vi "Untitled 2.vi"() -> ()   [LabVIEW 2020]
uses:
  <vilib>/gpm_packages/@cs/linked-list/Source/Linked List/Linked List/Linked List.lvclass
  C:/Program Files/National Instruments/LabVIEW 2020/vi.lib/gpm_packages/@cs/linked-list/Source/Linked List/ILinkedList/ILinked List.lvclass
  <vilib>/gpm_packages/@cs/persistence/source/CAML/CAML.lvclass
  C:/Program Files/National Instruments/LabVIEW 2020/vi.lib/gpm_packages/@cs/persistence/source/IPersist/IPersist.lvclass
  <vilib>/gpm_packages/@cs/persistence/source/XML/XML.lvclass
  <vilib>/gpm_packages/@cs/user-manager/Source/User Configuration Manager/User Configuration Manager.lvclass
  <vilib>/gpm_packages/@cs/user-manager/Source/SHA-1 Encryption/SHA-1.lvclass
  C:/Program Files/National Instruments/LabVIEW 2020/vi.lib/gpm_packages/@cs/user-manager/Source/iEncryption/iEncryption.lvclass
  <vilib>/gpm_packages/@cs/persistence/source/IPersist/IPersist.lvclass
  68168d1c-9d56-4a75-be37-98398c79d179.vi
  <vilib>/gpm_packages/@cs/linked-list/Source/Linked List/ILinkedList/ILinked List.lvclass
  <vilib>/gpm_packages/@cs/linked-list/Source/Linked List/Linked List Ref/Linked List Ref.lvclass
panel:
  out "error out 2":errorcluster
  out "error out":errorcluster
  out "Verification Message":string
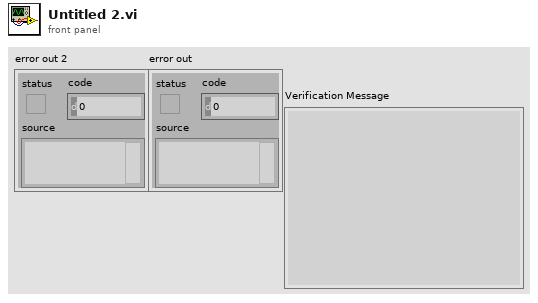
[diagram p1: front panel]
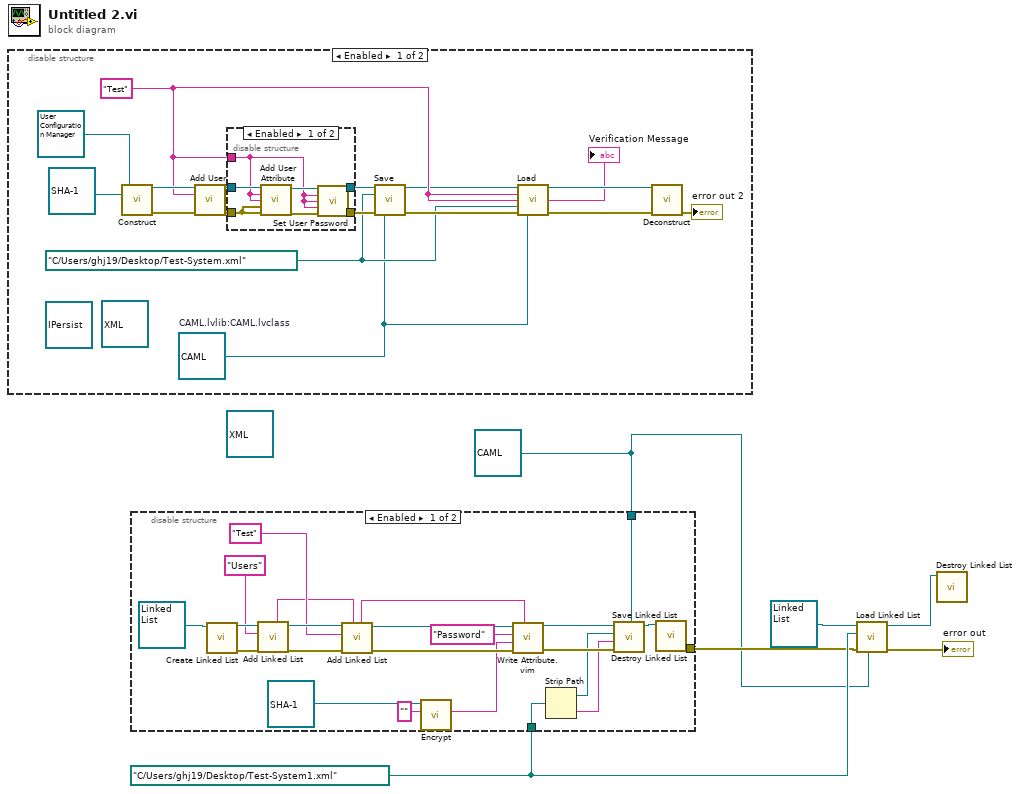
[diagram p0: block diagram]
diagram:
  w1 = refnum<class "CAML.lvclass"> refnum ("CAML.lvlib:CAML.lvclass")
  (unwired) refnum<class "XML.lvclass"> refnum ("XML.lvlib:XML.lvclass")
  w5 = path "C:/Users/ghj19/Desktop/Test-System1.xml"
  n1 = disable-structure shown="Enabled" {
    frame Enabled {
      w8 = refnum<class "CAML.lvclass"> refnum  # CAML.lvlib:CAML.lvclass
      (unwired) refnum<class "IPersist.lvclass"> refnum ("IPersist.lvlib:IPersist.lvclass")
      w10 = path "C:/Users/ghj19/Desktop/Test-System.xml"
      w16 = "Test" ("Username")
      (unwired) refnum<class "XML.lvclass"> refnum ("XML.lvlib:XML.lvclass")
      n2 = call-dynamic "Construct.vi"("User Configuration Manager in"=refnum<class "User Configuration Manager.lvclass"> refnum ("User Configuration Manager.lvlib:User Configuration Manager"), "Encryption Type"=refnum<class "SHA-1.lvclass"> refnum ("User Configuration Manager.lvlib:SHA-1.lvclass")) -> ("User Configuration Manager out"=w19:refnum<class "User Configuration Manager.lvclass">, "error out"=w18:errorcluster)  [unwired: 12 in]
      n3 = call-dynamic "Add User.vi"("User Configuration Manager in"=w19, "Username"=w16, "error in (no error)"=w18) -> ("User Configuration Manager out"=w17:refnum<class "User Configuration Manager.lvclass">, "error out"=w15:errorcluster)  [unwired: 10 in, 1 out]
      n4 = disable-structure shown="Enabled" {
        disable-tunnel: w17 -> [w30 w31]
        disable-tunnel: w16 -> [w28 _]
        disable-tunnel: w15 -> [w26 w32]
        disable-tunnel: [w25 w31] -> w13
        disable-tunnel: [w24 w32] -> w11
        frame Enabled {
          n5 = call-dynamic "Add User Attribute.vi"("User Configuration Manager in"=w30, "Username"=w28, "Attribute Name"=w28, "Attribute Value"=w26, "error in (no error)"=w26) -> ("User Configuration Manager out"=w29:refnum<class "User Configuration Manager.lvclass">, "error out"=w27:errorcluster)  [unwired: 8 in, 1 out]
          n6 = call-dynamic "Set User Password.vi"("User Configuration Manager in"=w29, "Username"=w28, "Current Password"=w28, "New Password"=w28, "error in (no error)"=w27) -> ("User Configuration Manager out"=w25:refnum<class "User Configuration Manager.lvclass">, "error out"=w24:errorcluster)  [unwired: 8 in, 1 out]
        }
        frame Disabled {
        }
      }
      n7 = call-dynamic "Save.vi"("User Configuration Manager in"=w13, "Path"=w10, "error in (no error)"=w11, "Persistence"=w8) -> ("User Configuration Manager out"=w9:refnum<class "User Configuration Manager.lvclass">, "error out"=w12:errorcluster)  [unwired: 10 in]
      n8 = call-dynamic "Load.vi"("User Configuration Manager"=w9, "Username"=w16, "Password"=w16, "Path"=w10, "error in (no error)"=w12, "Persistence"=w8) -> ("User Configuration Manager"=w21:refnum<class "User Configuration Manager.lvclass">, "Verification Message"=→"Verification Message":string, "error out"=w14:errorcluster)  [unwired: 6 in, 1 out]
      n9 = call-dynamic "Deconstruct.vi"("User Configuration Manager in"=w21, "error in (no error)"=w14) -> ("error out"=→"error out 2":errorcluster)  [unwired: 13 in]
    }
    frame Disabled {
    }
  }
  n10 = disable-structure shown="Enabled" {
    disable-tunnel: w5 -> [w41 _]
    disable-tunnel: w1 -> [w36 _]
    disable-tunnel: [w33 _] -> w3
    frame Enabled {
      n11 = call <vilib>:"Create Linked List.vi"("Linked List"=refnum<class "Linked List.lvclass"> refnum ("Linked Lists.lvlib:Linked List.lvclass")) -> ("error out"=w53:errorcluster, "Linked List Ref"=w55:refnum<data-value>)  [unwired: 9 in]
      n12 = call <vilib>:"Add Linked List.vi"("error in (no error)"=w53, "Name"="Users", "Linked List Ref"=w55) -> ("error out"=w39:errorcluster, "Linked List Ref out"=w49:refnum<data-value>, "Linked List ID out"=w35:string)  [unwired: 5 in, 1 out]
      n13 = call <vilib>:"Add Linked List.vi"("Parent ID"=w35, "error in (no error)"=w39, "Name"="Test", "Linked List Ref"=w49) -> ("error out"=w50:errorcluster, "Linked List Ref out"=w37:refnum<data-value>, "Linked List ID out"=w47:string)  [unwired: 4 in, 1 out]
      n14 = call-dynamic "Encrypt.vi"("String"="", "SHA-1 in"=refnum<class "SHA-1.lvclass"> refnum ("User Configuration Manager.lvlib:SHA-1.lvclass")) -> ("Encrypted String"=w38:string)  [unwired: 9 in]
      n15 = call "Write Attribute.vim"("Linked List ID"=w47, "error in (no error)"=w50, "Attribute"=w38, "Attribute Name"="Password", "Linked List Ref"=w37) -> ("error out"=w44:errorcluster, "Linked List Ref out"=w45:refnum<data-value>)  [unwired: 3 in, 2 out]
      n16 = Strip Path(path=w41) -> (stripped path=w43:path, name=w42:string)
      n17 = call <vilib>:"Save Linked List.vi"("Persistence"=w36, "error in (no error)"=w44, "File Name"=w42, "Folder"=w43, "Linked List Ref"=w45) -> ("Linked List Ref out"=w34:refnum<data-value>)  [unwired: 5 in, 1 out]
      n18 = call <vilib>:"Destroy Linked List.vi"("Linked List Ref"=w34) -> ("error out"=w33:errorcluster)  [unwired: 10 in]
    }
    frame Disabled {
    }
  }
  n19 = call <vilib>:"Load Linked List.vi"("Persistence"=w1, "error in (no error)"=w3, "File Path"=w5, "Linked List"=refnum<class "Linked List.lvclass"> refnum ("Linked Lists.lvlib:Linked List.lvclass")) -> ("error out"=→"error out":errorcluster, "Linked List Ref out"=w2:refnum<data-value>)  [unwired: 5 in, 1 out]
  n20 = call <vilib>:"Destroy Linked List.vi"("Linked List Ref"=w2) -> ()  [unwired: 10 in, 1 out]
